vi "windows_heater_safety.vi"(4 "Maximum Test Section Temperature":refnum<vi>, 5 "Stop!":refnum<vi>, 6 "Test Section Temperatures":refnum<vi>[](array[refnum]), 7 "Minimum Flow Rate Refnum":refnum<vi>, 8 "Liquid Flow Rate Refnum":refnum<vi>, 9 "Vapor Flow Rate Refnum":refnum<vi>, 10 "Safety Trigger Refnum":refnum<vi>, 11 "Switch Refnum":refnum<vi>) -> ()   [LabVIEW 2017]
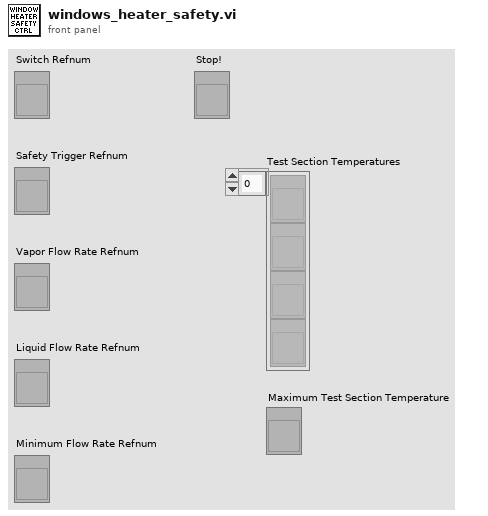
[diagram p1: front panel]
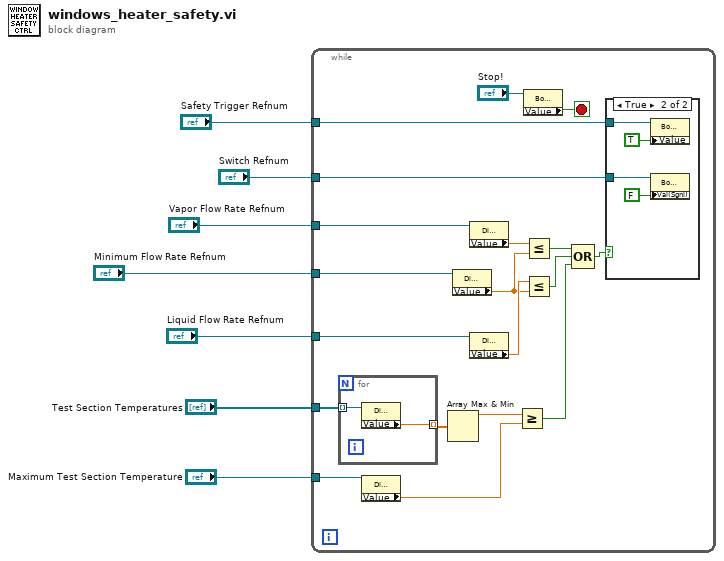
[diagram p0: block diagram]
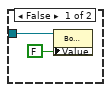
[diagram p2: hidden frame]
diagram:
  n1 = while {
    tunnel: "Vapor Flow Rate Refnum" -> [w26]
    tunnel: "Liquid Flow Rate Refnum" -> [w25]
    tunnel: "Switch Refnum" -> [w17]
    tunnel: "Safety Trigger Refnum" -> [w16]
    tunnel: "Minimum Flow Rate Refnum" -> [w15]
    tunnel: "Test Section Temperatures" -> [w13]
    tunnel: "Maximum Test Section Temperature" -> [w10]
    stop <- w19 stop-if-true
    n2 = for {
      tunnel: w13 -> [w28] mode=indexing
      tunnel: [w27] -> w12 mode=indexing
      n3 = property class="DigNum (strict)"(reference=w28) -> ("Value"=w27:dbl)  [unwired: 1 in, 2 out]
    }
    n4 = property class="DigNum (strict)"(reference=w10) -> ("Value"=w9:dbl)  [unwired: 1 in, 2 out]
    n5 = Array Max & Min(array=w12) -> (max value=w11:dbl)  [unwired: 3 out]
    n6 = property class="DigNum (strict)"(reference=w15) -> ("Value"=w14:dbl)  [unwired: 1 in, 2 out]
    n7 = property class="DigNum (strict)"(reference=w26) -> ("Value"=w24:dbl)  [unwired: 1 in, 2 out]
    n8 = property class="DigNum (strict)"(reference=w25) -> ("Value"=w23:dbl)  [unwired: 1 in, 2 out]
    n9 = Greater Or Equal?(x=w11, y=w9) -> (x >= y?=w8:bool)
    n10 = property class="Bool (strict)"(reference="Stop!") -> ("Value"=w19:bool)  [unwired: 1 in, 2 out]
    n11 = Less Or Equal?(x=w24, y=w14) -> (x <= y?=w22:bool)
    n12 = Less Or Equal?(x=w23, y=w14) -> (x <= y?=w21:bool)
    n13 = Compound Arithmetic op=OR(w22, w21, w8) -> (w18:bool)
    n14 = case shown="True" w18 {
      tunnel: w17 -> [_ w33]
      tunnel: w16 -> [w29 w31]
      frame False {
        n15 = property class="Bool (strict)"(reference=w29, "Value"=FALSE) -> ()  [unwired: 1 in, 2 out]
      }
      frame True {
        n16 = property class="Bool (strict)"(reference=w31, "Value"=TRUE) -> ()  [unwired: 1 in, 2 out]
        n17 = property class="Bool (strict)"(reference=w33, "Val(Sgnl)"=FALSE ("Value")) -> ()  [unwired: 1 in, 2 out]
      }
    }
  }
